vi "String Constant.vi"(8 "error in (no error)":errorcluster caption="错误输入（无错误）", 11 "Name":string) -> (0 "error out":errorcluster, 3 "Value":string)   [LabVIEW 2013, in "Resource Constant.lvlib"]
uses:
  Resource Constant.lvlib
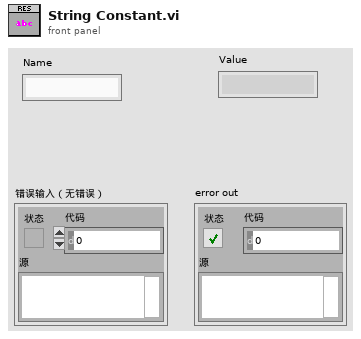
[diagram p1: front panel]
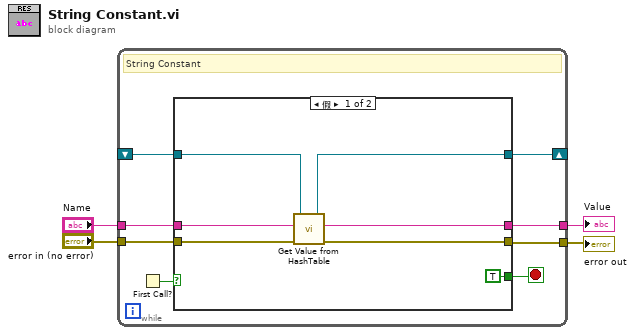
[diagram p0: block diagram]
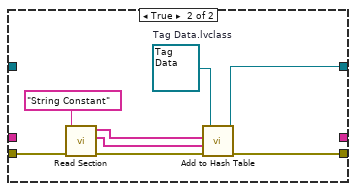
[diagram p2: hidden frame]
diagram:
  n1 = while {
    shift-right: [w9] -> _
    shift-left: _ -> [w8]
    tunnel: "error in (no error)" -> [w11]
    tunnel: [w10] -> w3
    tunnel: "Name" -> [w6]
    tunnel: [w5] -> w1
    stop <- w7 stop-if-true
    # "String Constant"
    n2 = First Call?() -> (First Call?: T/F=w12:bool)
    n3 = case shown="假" w12 {
      tunnel: w11 -> [w14 w23]
      tunnel: [w13 w21] -> w10
      tunnel: [w15 w20] -> w9
      tunnel: w8 -> [w18 _]
      tunnel: [TRUE _] -> w7
      tunnel: w6 -> [w17 _]
      tunnel: [w16 _] -> w5
      frame False {
        n4 = call-poly "Get Value from HashTable.vi"("error in (no error)"=w14, "Name"=w17, "Contstant Base 输入"=w18) -> ("error out"=w13:errorcluster, "Value"=w16:string, "Contstant Base 输出"=w15:refnum<class "Tag Data.lvclass">)  [unwired: 6 in]
      }
      frame True {
        w26 = refnum<class "Tag Data.lvclass"> refnum  # Tag Data.lvclass
        n5 = call "Read Section.vi"("error in (no error)"=w23, "section"="String Constant") -> ("error out"=w22:errorcluster, "Value"=w24:string[], "key names"=w25:string[])  [unwired: 7 in]
        n6 = call-poly "Add to Hash Table.vi"("error in (no error)"=w22, "Value"=w24, "Name"=w25, "Contstant Base 输入"=w26) -> ("error out"=w21:errorcluster, "Contstant Base 输出"=w20:refnum<class "Tag Data.lvclass">)  [unwired: 6 in]
      }
    }
  }
  "error out" <- w3
  "Value" <- w1
